vi "DC_OUTPUT.vi"(0 "String":string, 1 "Current Output [A]":dbl(knob) scale=0.0..1.0, 2 "Voltage Output [V]":dbl(knob) scale=12.0..15.0) -> ()   [LabVIEW 2019]
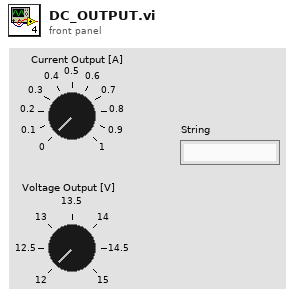
[diagram p1: front panel]
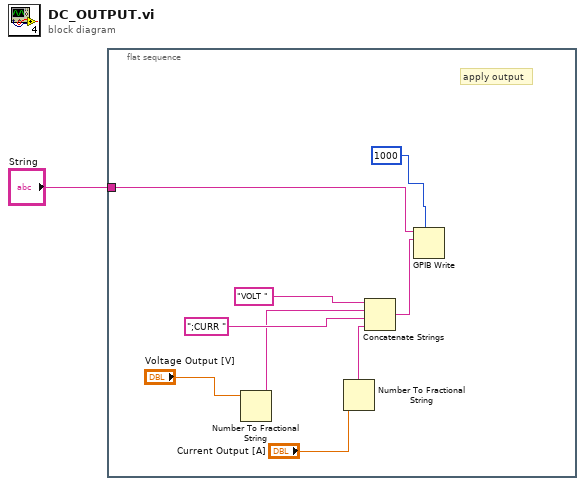
[diagram p0: block diagram]
diagram:
  n1 = flat-sequence {
    tunnel: "String" -> [w2]
    frame #0 {
      # "apply output"
      n2 = Number To Fractional String(number="Voltage Output [V]") -> (F-format string=w8:string)  [unwired: 3 in]
      n3 = Number To Fractional String(number="Current Output [A]") -> (F-format string=w7:string)  [unwired: 3 in]
      n4 = Concatenate Strings("VOLT " ("data"), w8, ";CURR " ("data"), w7) -> (w6:string)
      n5 = GPIB Write(0:w2, 1:w6, 4:1000) -> ()  [unwired: 2 in, 2 out]
    }
  }
